vi "Fieldscan - save data to file.vi"(8 "error in (no error)":errorcluster, 10 "Data":T1, 11 "Action":T2) -> (0 "error out":errorcluster, 3 "File path":path)   [LabVIEW 2019]
doc: "Nicolas Weiss - EPFL - IPHYS 2019\n----"
uses:
  Controls/Save data file action.ctl
  Controls/Data to save cluster.ctl
  Controls/Log destination selector.ctl
  _Global variables 1.vi
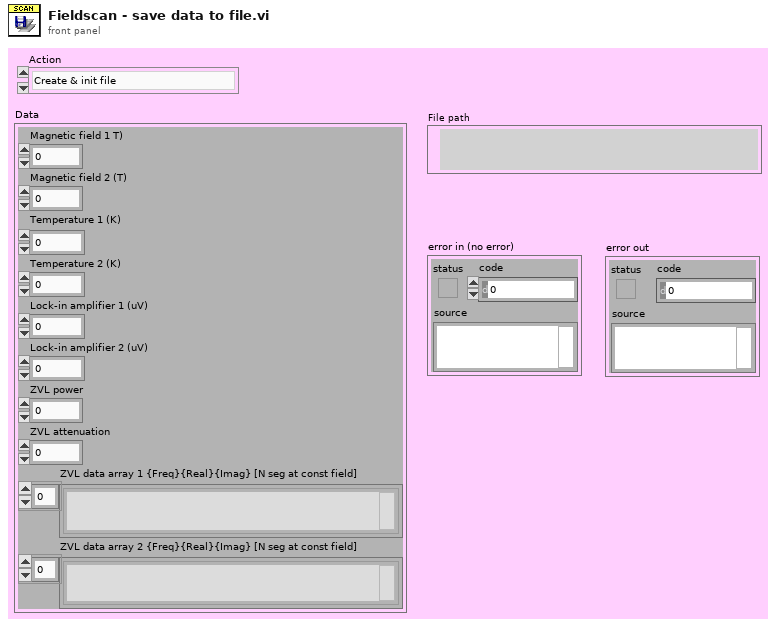
[diagram p1: front panel]
types:
  T1 = typedef "Data to save cluster.ctl" = cluster{"Magnetic field 1 T)":dbl, "Magnetic field 2 (T)":dbl, "Temperature 1 (K)":dbl, "Temperature 2 (K)":dbl, "Lock-in amplifier 1 (uV)":dbl, "Lock-in amplifier 2 (uV)":dbl, "ZVL power":dbl, "ZVL attenuation":dbl, "ZVL data array 1 {Freq}{Real}{Imag} [N seg at const field]":string[], "ZVL data array 2 {Freq}{Real}{Imag} [N seg at const field]":string[]}
  T2 = typedef "Save data file action.ctl" = enum16{"Create & init file", "Append data", "Close file"}
  T3 = typedef "Log destination selector.ctl" = enum16{"UI", "File", "UI+file"}
  T4 = enum16{"open", "replace", "create", "open or create", "replace or create", "replace or create with confirmation"}
  T5 = cluster{"Magnetic field 1 T)":dbl, "Magnetic field 2 (T)":dbl}
  T6 = cluster{"Temperature 1 (K)":dbl, "Temperature 2 (K)":dbl}
  T7 = cluster{"Lock-in amplifier 1 (uV)":dbl, "Lock-in amplifier 2 (uV)":dbl}
  T8 = cluster{"ZVL power":dbl, "ZVL attenuation":dbl, "Data":string, "Data":string}
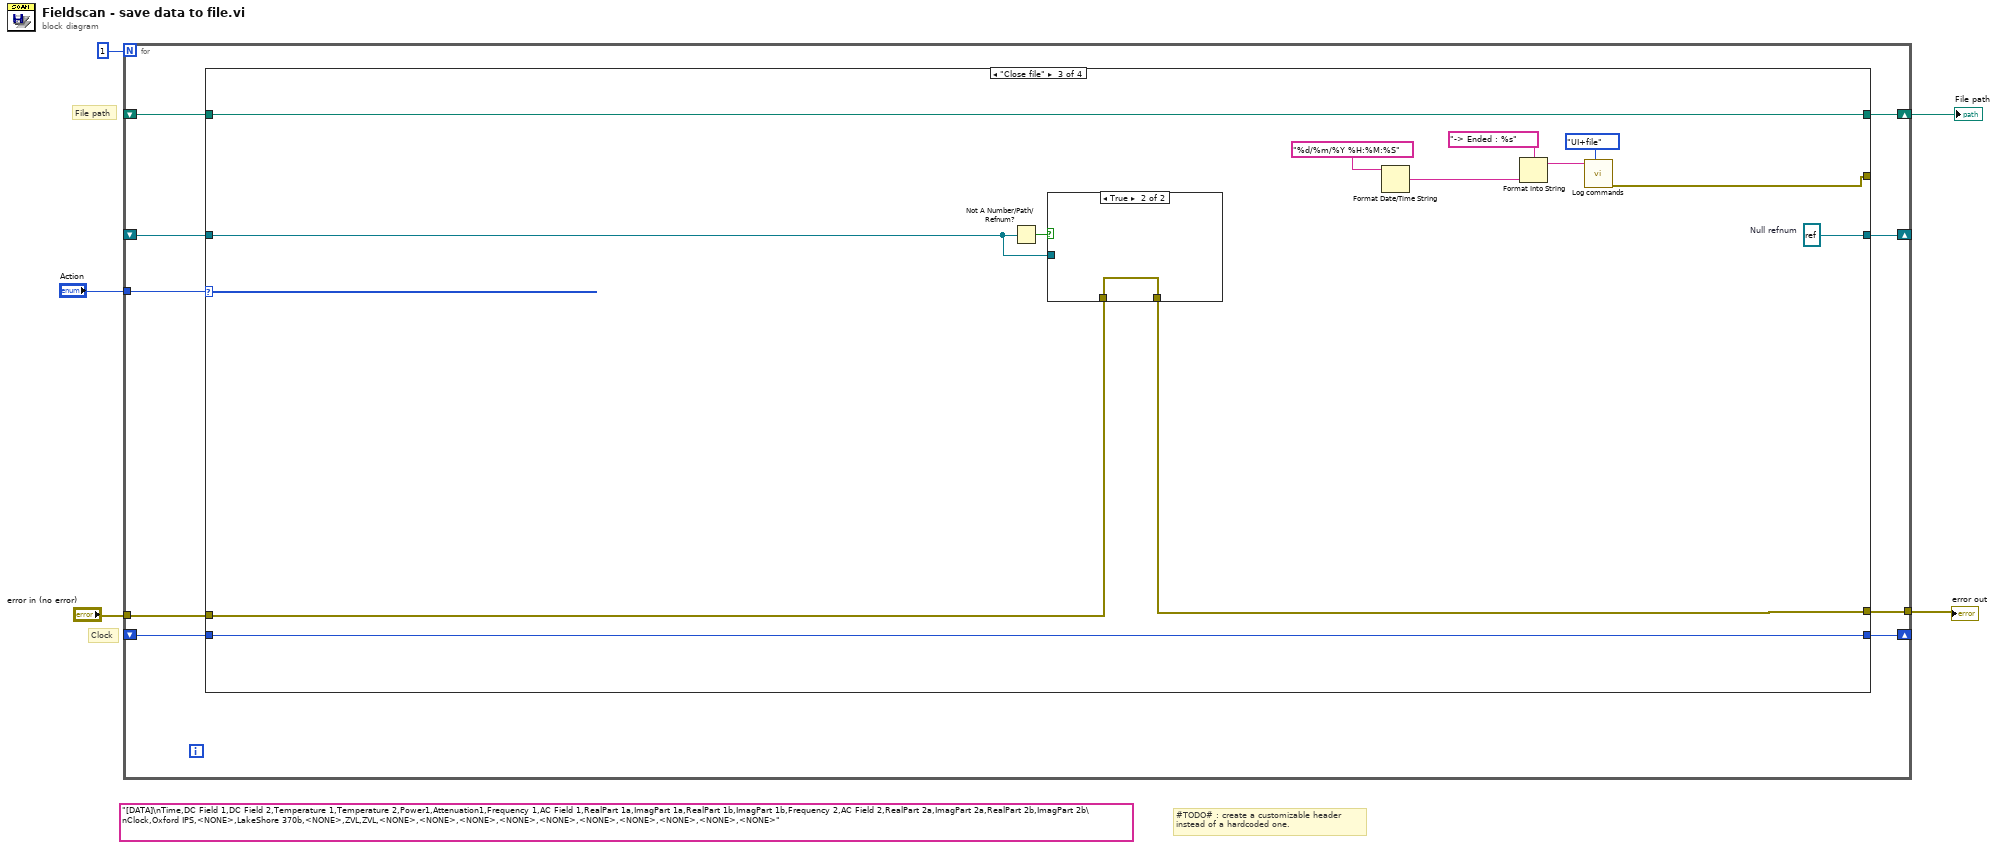
[diagram p0: block diagram]
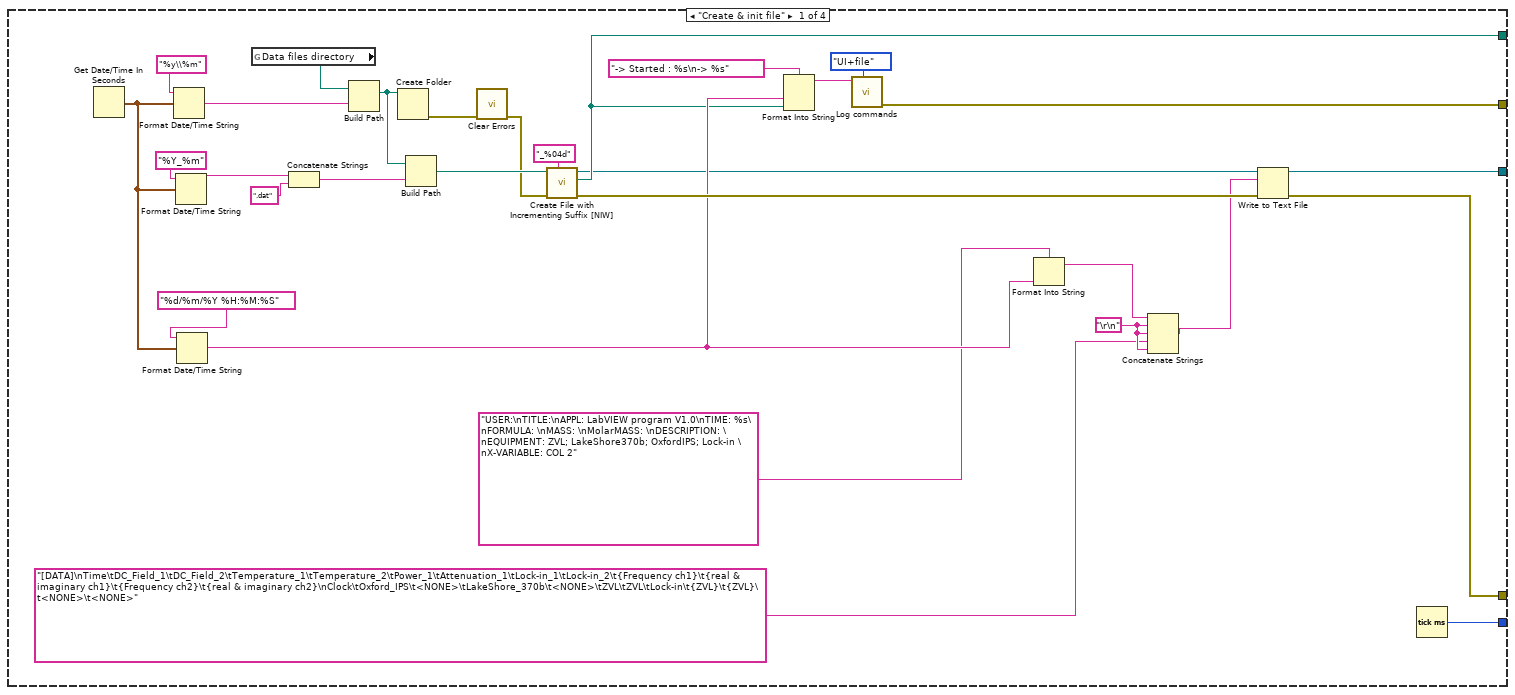
[diagram p2: hidden frame]
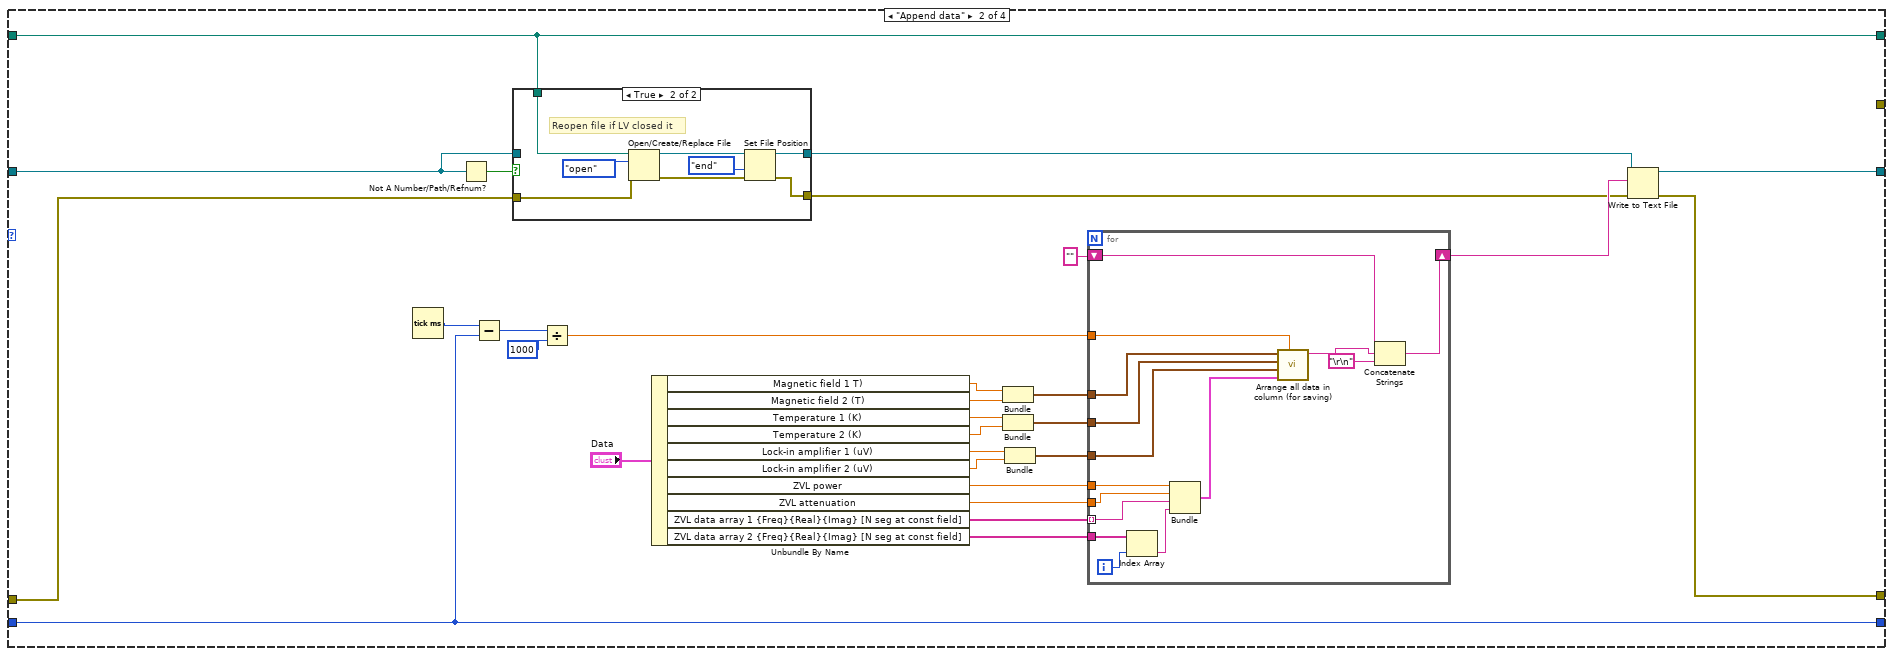
[diagram p3: hidden frame]
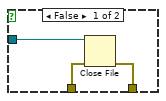
[diagram p5: hidden frame]
diagram:
  (unwired) "[DATA]\nTime,DC Field 1,DC Field 2,Temperature 1,Temperature 2,Power1,Attenuation1,Frequency 1,AC Field 1,RealPart 1a,ImagPart 1a,RealPart 1b,ImagPart 1b,Frequency 2,AC Field 2,RealPart 2a,ImagPart 2a,RealPart 2b,ImagPart 2b\nClock,Oxford IPS,<NONE>,LakeShore 370b,<NONE>,ZVL,ZVL,<NONE>,<NONE>,<NONE>,<NONE>,<NONE>,<NONE>,<NONE>,<NONE>,<NONE>,<NONE>" ("time format string (%c)")
  # "File path"
  # "Clock"
  # "#TODO# : create a customizable header \ninstead of a hardcoded one."
  n1 = for {
    N: 1 -> [_]
    shift-right: [w14] -> _
    shift-left: _ -> [w6]
    tunnel: "Action" -> [w13]
    tunnel: "error in (no error)" -> [w12]
    tunnel: [w11] -> w2
    shift-right: [w9] -> _
    shift-left: _ -> [w10]
    shift-right: [w8] -> w1
    shift-left: _ -> [w7]
    n2 = case shown="\"Close file\"" w13 {
      tunnel: [w18 w73 w106 w117] -> w14
      tunnel: w6 -> [_ w61 w99 w117]
      tunnel: w12 -> [_ w60 w111 w116]
      tunnel: [w34 w66 w110 w116] -> w11
      tunnel: w10 -> [_ w71 w102 w118]
      tunnel: [w28 w71 w102 w118] -> w9
      tunnel: [w23 w64 w103 w119] -> w8
      tunnel: w7 -> [_ w64 w103 w119]
      tunnel: [w19 _ w101 _] -> _
      frame "Create & init file" {
        w29 = "\r\n"
        n3 = Get Date/Time In Seconds() -> (seconds since 1Jan1904=w33:timestamp)
        n4 = Format Date/Time String(time format string (%c)="%y\\%m", seconds (now)=w33) -> (date/time string=w43:string)  [unwired: 1 in]
        n5 = Format Date/Time String(time format string (%c)="%Y_%m", seconds (now)=w33) -> (date/time string=w38:string)  [unwired: 1 in]
        n6 = Format Date/Time String(time format string (%c)="%d/%m/%Y %H:%M:%S", seconds (now)=w33) -> (date/time string=w26:string)  [unwired: 1 in]
        n7 = global read "_Global variables 1.vi" "Data files directory"() -> (w16:path)
        n8 = Concatenate Strings(w38, ".dat" ("string")) -> (w36:string)
        n9 = Build Path(base path=w16, name or relative path=w43) -> (appended path=w42:path)
        n10 = Create Folder(path (use dialog)=w42) -> (error out=w22:errorcluster)  [unwired: 2 in, 2 out]
        n11 = Build Path(base path=w42, name or relative path=w36) -> (appended path=w41:path)
        n12 = call <vilib>:"Clear Errors.vi"("error in (no error)"=w22) -> ("error out"=w21:errorcluster)  [unwired: 5 in, 1 out]
        n13 = call "Create File with Incrementing Suffix [NIW].vi"("format string (\" (%03d)\")"="_%04d" ("format string (\" (%03d)\")"), "error in (no error)"=w21, "file path"=w41) -> ("error out"=w35:errorcluster, "actual path"=w23:path, "refnum out"=w20:refnum<file>)  [unwired: 5 in, 1 out]
        n14 = Format Into String(format string="-> Started : %s\n-> %s" ("string"), w26, w23) -> (resulting string=w25:string)  [unwired: 2 in, 1 out]
        n15 = call "Log commands.vi"("Log destination"=Log_destination_selector."UI+file", "text to log"=w25) -> ("error out"=w19:errorcluster)  [unwired: 9 in]
        n16 = Format Into String(format string="USER:\nTITLE:\nAPPL: LabVIEW program V1.0\nTIME: %s\nFORMULA: \nMASS: \nMolarMASS: \nDESCRIPTION: \nEQUIPMENT: ZVL; LakeShore370b; OxfordIPS; Lock-in \nX-VARIABLE: COL 2" ("time format string (%c)"), w26) -> (resulting string=w30:string)  [unwired: 2 in, 1 out]
        n17 = Concatenate Strings(w30, w29, w29, "[DATA]\nTime\tDC_Field_1\tDC_Field_2\tTemperature_1\tTemperature_2\tPower_1\tAttenuation_1\tLock-in_1\tLock-in_2\t{Frequency ch1}\t{real & imaginary ch1}\t{Frequency ch2}\t{real & imaginary ch2}\nClock\tOxford_IPS\t<NONE>\tLakeShore_370b\t<NONE>\tZVL\tZVL\tLock-in\t{ZVL}\t{ZVL}\t<NONE>\t<NONE>" ("time format string (%c)"), w29) -> (w31:string)
        n18 = Write to Text File(file (use dialog)=w20, text=w31, error in=w35) -> (refnum out=w18:refnum<file>, error out=w34:errorcluster)  [unwired: 1 in, 1 out]
        n19 = Tick Count (ms)() -> (millisecond timer value=w28:u32)
      }
      frame "Append data" {
        n20 = Tick Count (ms)() -> (millisecond timer value=w72:u32)
        n21 = Not A Number/Path/Refnum?(number/path/refnum=w61) -> (NaN/Path/Refnum?=w65:bool)
        n22 = Subtract(x=w72, y=w71) -> (x-y=w70:u32)
        n23 = case shown="True" w65 {
          tunnel: w64 -> [_ w82]
          tunnel: [w75 w76] -> w63
          tunnel: w61 -> [w75 _]
          tunnel: w60 -> [w74 w81]
          tunnel: [w74 w77] -> w59
          frame False {
          }
          frame True {
            # "Reopen file if LV closed it"
            n24 = Open/Create/Replace File(file path (use dialog)=w82, error in=w81, operation (0:open)=T4."open") -> (refnum out=w80:refnum<file>, error out=w78:errorcluster)  [unwired: 3 in, 1 out]
            n25 = Set File Position(refnum=w80, from (0:start)=enum16{"start", "end", "current"}."end", error in=w78) -> (refnum out=w76:refnum<file>, error out=w77:errorcluster)  [unwired: 1 in]
          }
        }
        n26 = Divide(x=w70, y=u32 1000 ("x")) -> (x/y=w68:dbl)
        n27 = Unbundle By Name("Data") -> ("Magnetic field 1 T)"=w56:dbl, "Magnetic field 2 (T)"=w57:dbl, "Temperature 1 (K)"=w54:dbl, "Temperature 2 (K)"=w53:dbl, "Lock-in amplifier 1 (uV)"=w51:dbl, "Lock-in amplifier 2 (uV)"=w50:dbl, "ZVL power"=w48:dbl, "ZVL attenuation"=w47:dbl, "ZVL data array 1 {Freq}{Real}{Imag} [N seg at const field]"=w46:string[], "ZVL data array 2 {Freq}{Real}{Imag} [N seg at const field]"=w45:string[])
        n28 = Bundle("Magnetic field 1 T)"=w56, "Magnetic field 2 (T)"=w57) -> (w55:T5)  [unwired: 1 in]
        n29 = Bundle("Temperature 1 (K)"=w54, "Temperature 2 (K)"=w53) -> (w52:T6)  [unwired: 1 in]
        n30 = Bundle("Lock-in amplifier 1 (uV)"=w51, "Lock-in amplifier 2 (uV)"=w50) -> (w49:T7)  [unwired: 1 in]
        n31 = for {
          tunnel: w68 -> [w95]
          shift-right: [w97] -> w62
          shift-left: "" ("ZVL data 2 [1 segment]") -> [w96]
          tunnel: w55 -> [w93]
          tunnel: w52 -> [w92]
          tunnel: w49 -> [w91]
          tunnel: w48 -> [w90]
          tunnel: w47 -> [w89]
          tunnel: w46 -> [w88] mode=indexing
          tunnel: w45 -> [w86]
          i -> [w87]
          n32 = Index Array(array=w86, index=w87) -> (element=w85:string)
          n33 = Bundle("ZVL power"=w90, "ZVL attenuation"=w89, "Data"=w88, "Data"=w85) -> (w84:T8)  [unwired: 1 in]
          n34 = call "Arrange all data in column (for saving).vi"("Time (s)"=w95, "ZVL"=w84, "Lock-in Amplifier"=w91, "Lakeshore"=w92, "Magnetic field"=w93) -> ("Result string (for saving)"=w94:string)  [unwired: 6 in]
          n35 = Concatenate Strings(w96, w94, "\r\n") -> (w97:string)
        }
        n36 = Write to Text File(file (use dialog)=w63, text=w62, error in=w59) -> (refnum out=w73:refnum<file>, error out=w66:errorcluster)  [unwired: 1 in, 1 out]
      }
      frame "Close file" {
        w106 = refnum<file> refnum  # Null refnum
        n37 = Not A Number/Path/Refnum?(number/path/refnum=w99) -> (NaN/Path/Refnum?=w100:bool)
        n38 = case shown="True" w100 {
          tunnel: w111 -> [w114 w115]
          tunnel: [w113 w115] -> w110
          tunnel: w99 -> [w112 _]
          frame False {
            n39 = Close File(refnum=w112, error in=w114) -> (error out=w113:errorcluster)  [unwired: 1 out]
          }
          frame True {
          }
        }
        n40 = Format Date/Time String(time format string (%c)="%d/%m/%Y %H:%M:%S") -> (date/time string=w107:string)  [unwired: 2 in]
        n41 = Format Into String(format string="-> Ended : %s" ("string"), w107) -> (resulting string=w105:string)  [unwired: 2 in, 1 out]
        n42 = call "Log commands.vi"("Log destination"=Log_destination_selector."UI+file", "text to log"=w105) -> ("error out"=w101:errorcluster)  [unwired: 9 in]
      }
      frame Default {
        # "No Operation"
      }
    }
  }
  "error out" <- w2
  "File path" <- w1
